vi "vfh_explode_points.vi"(1 "VFH Resolution (Degrees)":i32, 2 "Resolution (meters)":dbl, 3 "Vehicle Radius (meters)":dbl=0.762, 4 "Distance":dbl) -> (0 "Exploded Iterations":dbl)   [LabVIEW 2010]
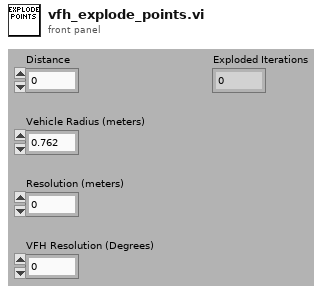
[diagram p1: front panel]
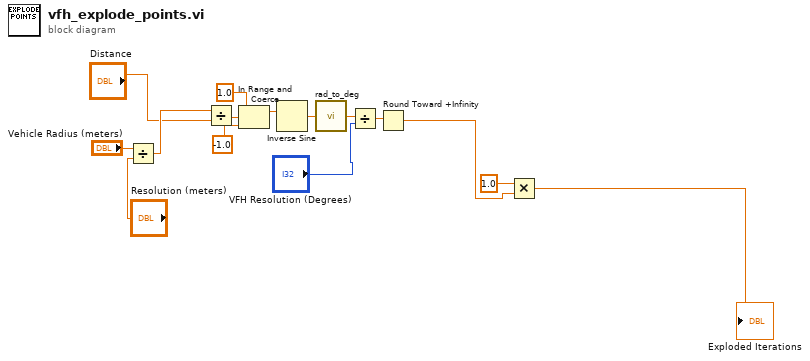
[diagram p0: block diagram]
diagram:
  n1 = Divide(x="Vehicle Radius (meters)", y="Resolution (meters)") -> (x/y=w3:dbl)
  n2 = Divide(x=w3, y="Distance") -> (x/y=w5:dbl)
  n3 = In Range and Coerce(upper limit=1.0, x=w5, lower limit=-1.0 ("upper limit")) -> (coerced(x)=w6:dbl)  [unwired: 1 out]
  n4 = Inverse Sine(1:w6) -> (0:w9:dbl)
  n5 = call "rad_to_deg.vi"("Radians"=w9) -> ("Degrees"=w10:dbl)
  n6 = Divide(x=w10, y="VFH Resolution (Degrees)") -> (x/y=w12:dbl)
  n7 = Round Toward +Infinity(x=w12) -> (ceil(x): smallest int >= x=w14:dbl)
  n8 = Multiply(x=1.0, y=w14) -> (x*y=→"Exploded Iterations":dbl)
